vi "Launch Connection Handlers.vi"(8 "error in (no error)":errorcluster, 11 "Server in":refnum<class "Server.lvclass">) -> (0 "error out":errorcluster, 3 "Server out":refnum<class "Server.lvclass">)   [LabVIEW 2013, in "MQTT Server.lvlib" / "Server.lvclass"]
uses:
  Server.lvclass
  Server.lvclass/Server.ctl
  MQTT_Base/Base Class/MQTT_Base.lvclass/MQTT_Base.ctl
  <vilib>/LabVIEW Open Source Project/MQTT Control Packets/Control Packets/ControlPacket/ControlPacket.lvclass
  MQTT_TCP/ConnectionHandler/TCPConnectionHandler.lvclass
  MQTT_Base/Base Class/MQTT_Base.lvclass
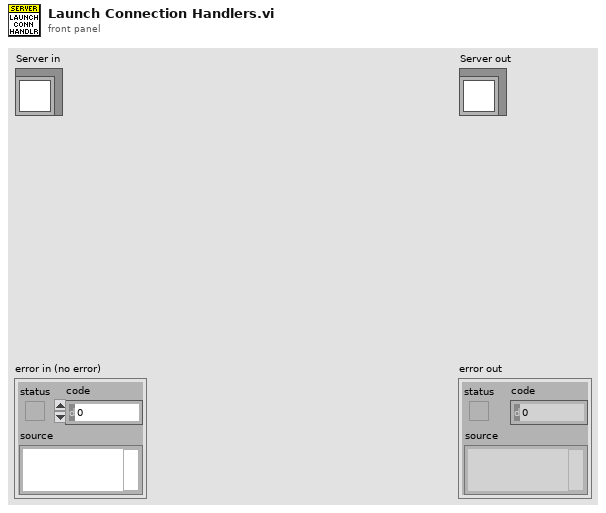
[diagram p1: front panel]
types:
  T1 = typedef "MQTT Server.lvlib/Server.lvclass/Public Events -- cluster.ctl" = cluster{"NbConnections":refnum<user-event>}
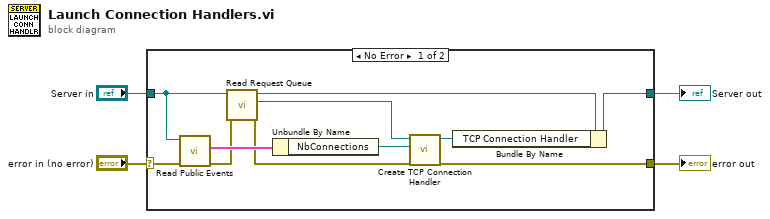
[diagram p0: block diagram]
diagram:
  n1 = case shown="No Error" "error in (no error)" {
    selector: "error in (no error)" -> [w7 w17]
    tunnel: [w11 w17] -> w3
    tunnel: [w15 w16] -> w1
    tunnel: "Server in" -> [w10 w16]
    frame No Error {
      n2 = call "Read Public Events.vi"("error in (no error)"=w7, "Server in"=w10) -> ("error out"=w6:errorcluster, "MQTT Server.Public Events"=w13:T1)  [unwired: 7 in, 1 out]
      n3 = call "Read Request Queue.vi"("error in (no error)"=w6, "MQTT_Base in"=w10) -> ("error out"=w5:errorcluster, "Request"=w8:refnum<queue>, "MQTT_Base out"=w9:refnum<class "Server.lvclass">)  [unwired: 7 in]
      n4 = Unbundle By Name(w13) -> ("NbConnections"=w12:refnum<user-event>)
      n5 = call "Create TCP Connection Handler.vi"("error in (no error)"=w5, "NbConnections"=w12, "ServerRequest"=w8) -> ("error out"=w11:errorcluster, "TCPConnectionHandler out"=w14:refnum<class "TCPConnectionHandler.lvclass">)  [unwired: 7 in]
      n6 = Bundle By Name(cluster=w9, "TCP Connection Handler"=w14) -> (w15:refnum<class "Server.lvclass">)
    }
    frame Error {
    }
  }
  "error out" <- w3
  "Server out" <- w1
